vi "IR_OPO_Capture_V2.vi"(0 "Commands array":string[][](array[string])=[["Group20.825", "Group20.671", "Group20.814", "Group30.121"], ["Group2-0.528", "Group2-1.243", "Group2-0.539", "Group30.121"], ["Group20.374", "Group21.573", "Group20.363", "Group30.121"], ["Group2-0.242", "Group2-1.815", "Group2-0.253", "Group30.121"], ["Group20.165", "Group21.991", "Group20.154", "Group30.121"], ["Group2-0.077", "Group2-2.145", "Group2-0.088", "Group30.121"], ["Group20.044", "Group22.233", "Group20.033", "Group30.121"], ["Group2-2.310", "WT10", "WT10", "Group30.121"], ["Group22.310", "WT10", "WT10", "Group30.121"], ["Group2-2.310", "WT10", "WT10", "Group30.121"], ["Group22.310", "WT10", "WT10", "Group30.121"], ["Group2-2.310", "WT10", "WT10", "Group30.121"], ["Group22.310", "WT10", "WT10", "Group30.121"], ["Group2-0.011", "Group2-2.277", "Group2-0.022", "Group30.121"], ["Group20.066", "Group22.189", "Group20.055", "Group30.121"], ["Group2-0.121", "Group2-2.057", "Group2-0.132", "Group30.121"], ["Group20.209", "Group21.903", "Group20.198", "Group30.121"], ["Group2-0.297", "Group2-1.705", "Group2-0.308", "Group30.121"], ["Group20.451", "Group21.419", "Group20.440", "Group30.121"], ["Group2-0.660", "Group2-0.979", "Group2-0.671", "Group30.121"]], 1 "Laser on/off array":bool[][](array[boolean])=[[FALSE, TRUE, FALSE, FALSE], [FALSE, TRUE, FALSE, FALSE], [FALSE, TRUE, FALSE, FALSE], [FALSE, TRUE, FALSE, FALSE], [FALSE, TRUE, FALSE, FALSE], [FALSE, TRUE, FALSE, FALSE], [FALSE, TRUE, FALSE, FALSE], [TRUE, FALSE, FALSE, FALSE], [TRUE, FALSE, FALSE, FALSE], [TRUE, FALSE, FALSE, FALSE], [TRUE, FALSE, FALSE, FALSE], [TRUE, FALSE, FALSE, FALSE], [TRUE, FALSE, FALSE, FALSE], [FALSE, TRUE, FALSE, FALSE], [FALSE, TRUE, FALSE, FALSE], [FALSE, TRUE, FALSE, FALSE], [FALSE, TRUE, FALSE, FALSE], [FALSE, TRUE, FALSE, FALSE], [FALSE, TRUE, FALSE, FALSE], [FALSE, TRUE, FALSE, FALSE]], 3 "AD status":bool, 4 "Axis 2":string="Group3", 5 "XPS_Address":string="192.168.254.254", 6 "Axis 1":string="Group2", 7 "laser array index":i32, 8 "OPO on?":bool, 9 "Process time":dbl format="%#_13g", 11 "Axis Speed":dbl=1.0 format="%#_13g", 12 "stop":bool, 13 "Axis Initial Parameters":T1={"Velocity (units/seconds)"=1.0, "Acceleration (units/seconds²)"=20.0, "Minimum Jerk Time (seconds)"=0.005, "Maximum Jerk Time (seconds)"=0.009} {"Maximum Jerk Time (seconds)" format="%.6e"; "Minimum Jerk Time (seconds)" format="%.6e"; "Acceleration (units/seconds²)" format="%.6e"; "Velocity (units/seconds)" format="%.6e"}, 14 "ROI Area \n(mm2)":dbl=4.035870075999999, 15 "Acceleration (units/seconds²)":dbl=20.0) -> (2 "Elapsed time":dbl)   [LabVIEW 2016]
uses:
  case selector.ctl
panel:
  out "Capture Log":string
  out "Axis 1 position":dbl format="%.10f"
  out "Axis 2 position":dbl format="%.10f"
  out "Initial time":timestamp
  in  "Active Positioner":string
  out "Current Line":i32
  out "1D Laser Array":bool[](array[boolean])=[FALSE, TRUE, FALSE, FALSE, FALSE, TRUE, FALSE, FALSE, FALSE, TRUE, FALSE, FALSE, FALSE, TRUE, FALSE, FALSE, FALSE, TRUE, FALSE, FALSE, FALSE, TRUE, FALSE, FALSE, FALSE, TRUE, FALSE, FALSE, TRUE, FALSE, FALSE, FALSE, TRUE, FALSE, FALSE, FALSE, TRUE, FALSE, FALSE, FALSE, TRUE, FALSE, FALSE, FALSE, TRUE, FALSE, FALSE, FALSE, TRUE, FALSE, FALSE, FALSE, FALSE, TRUE, FALSE, FALSE, FALSE, TRUE, FALSE, FALSE, FALSE, TRUE, FALSE, FALSE, FALSE, TRUE, FALSE, FALSE, FALSE, TRUE, FALSE, FALSE, FALSE, TRUE, FALSE, FALSE, FALSE, TRUE, FALSE, FALSE]
  out "1D command array":string[](array[string])=["Group20.825", "Group20.671", "Group20.814", "Group30.121", "Group2-0.528", "Group2-1.243", "Group2-0.539", "Group30.121", "Group20.374", "Group21.573", "Group20.363", "Group30.121", "Group2-0.242", "Group2-1.815", "Group2-0.253", "Group30.121", "Group20.165", "Group21.991", "Group20.154", "Group30.121", "Group2-0.077", "Group2-2.145", "Group2-0.088", "Group30.121", "Group20.044", "Group22.233", "Group20.033", "Group30.121", "Group2-2.310", "WT10", "WT10", "Group30.121", "Group22.310", "WT10", "WT10", "Group30.121", "Group2-2.310", "WT10", "WT10", "Group30.121", "Group22.310", "WT10", "WT10", "Group30.121", "Group2-2.310", "WT10", "WT10", "Group30.121", "Group22.310", "WT10", "WT10", "Group30.121", "Group2-0.011", "Group2-2.277", "Group2-0.022", "Group30.121", "Group20.066", "Group22.189", "Group20.055", "Group30.121", "Group2-0.121", "Group2-2.057", "Group2-0.132", "Group30.121", "Group20.209", "Group21.903", "Group20.198", "Group30.121", "Group2-0.297", "Group2-1.705", "Group2-0.308", "Group30.121", "Group20.451", "Group21.419", "Group20.440", "Group30.121", "Group2-0.660", "Group2-0.979", "Group2-0.671", "Group30.121"]
  out "Current Command":string
  out "Current laser element":bool
  out "Total lines":i32=80
  in  "Active Axis":string
  out "Laser on/off":bool
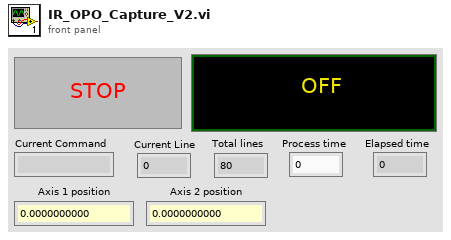
[diagram p1: front panel]
types:
  T1 = cluster{"Velocity (units/seconds)":dbl, "Acceleration (units/seconds²)":dbl, "Minimum Jerk Time (seconds)":dbl, "Maximum Jerk Time (seconds)":dbl}
  T2 = typedef "case selector.ctl" = enum16{"Initialize", "Element selection", "Laser", "Velocities", "Command", "Wait", "Exit"}
  T3 = enum16{"Initialize", "Lamp ON", "Lamp OFF", "Q-switch ON", "Q-switch OFF", "Adjust Energy", "Change Rep. Rate", "Send String"}
  T4 = enum16{"open", "replace", "create", "open or create", "replace or create", "replace or create with confirmation"}
  T5 = cluster{"connection TCP":refnum<k5>, "LogTo File":bool, "Log File refnum":refnum<file>, "no error if error log":bool}
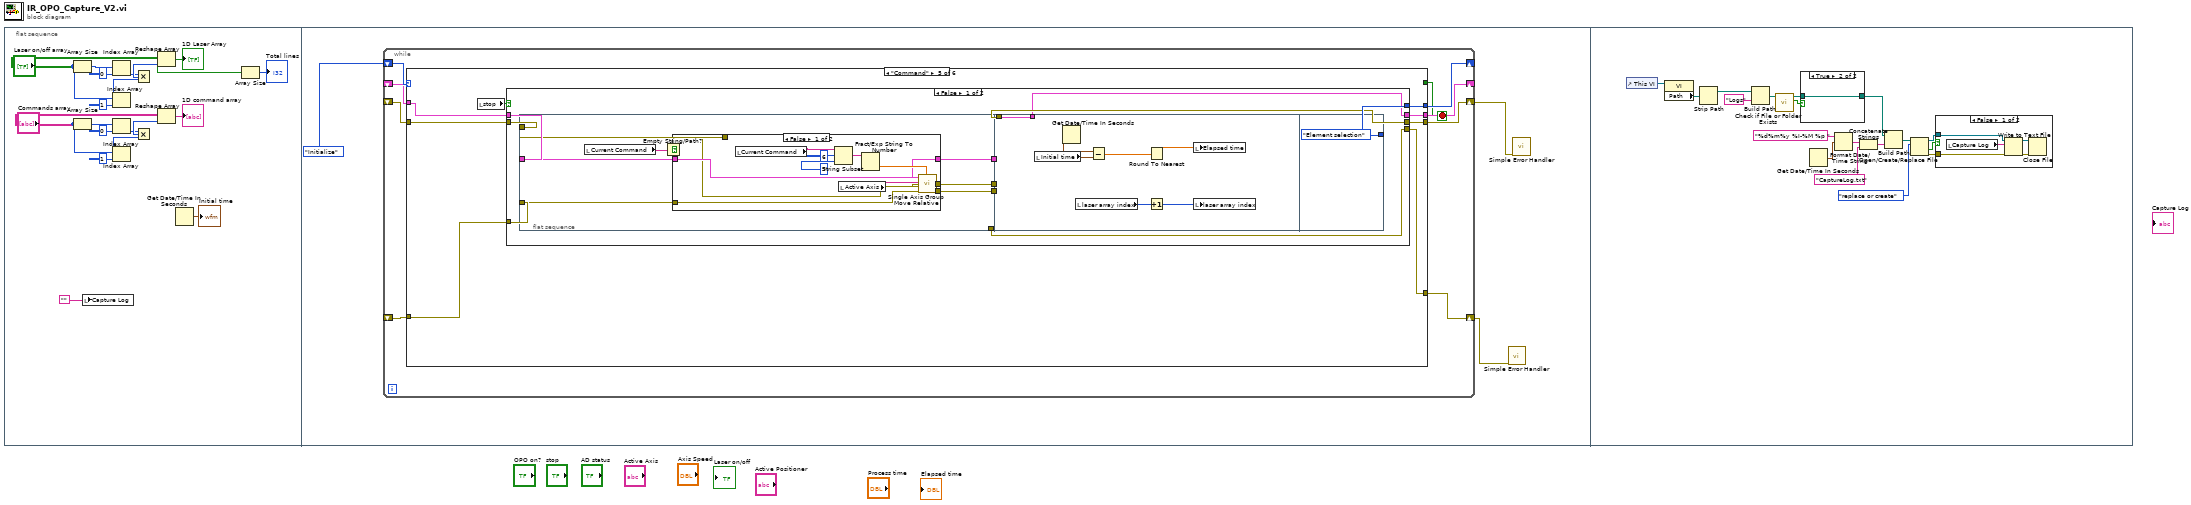
[diagram p0: block diagram]
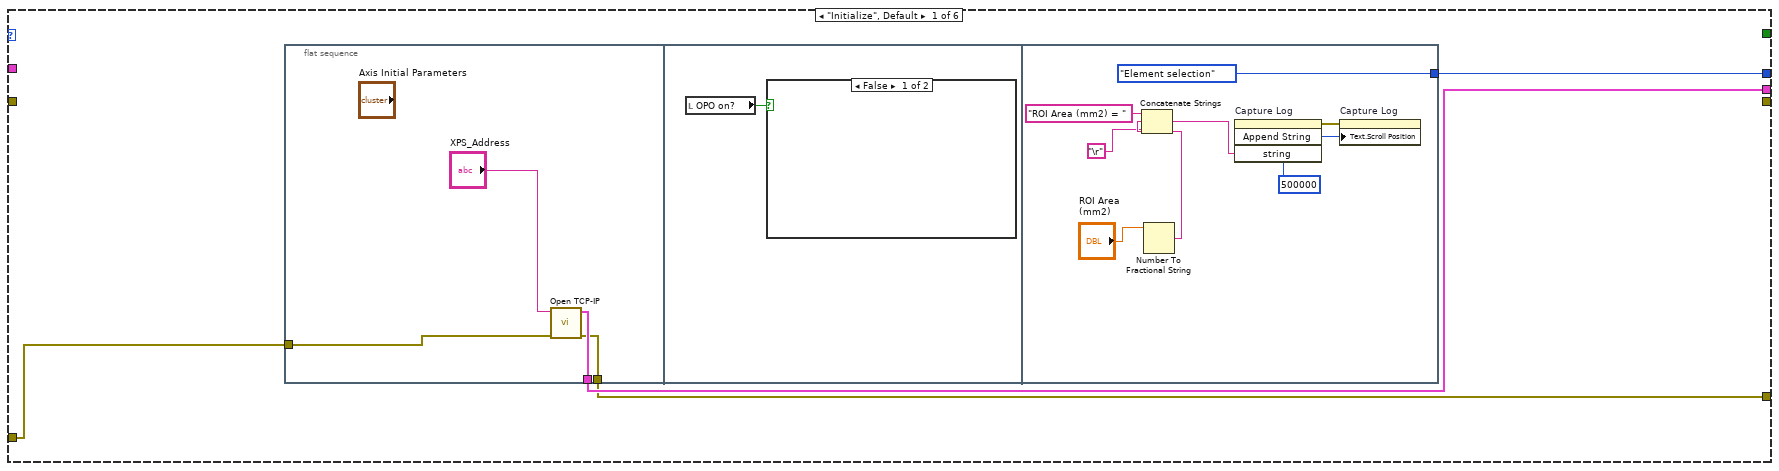
[diagram p2: hidden frame]
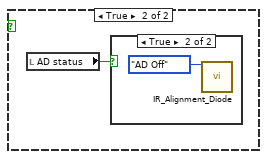
[diagram p3: hidden frame]
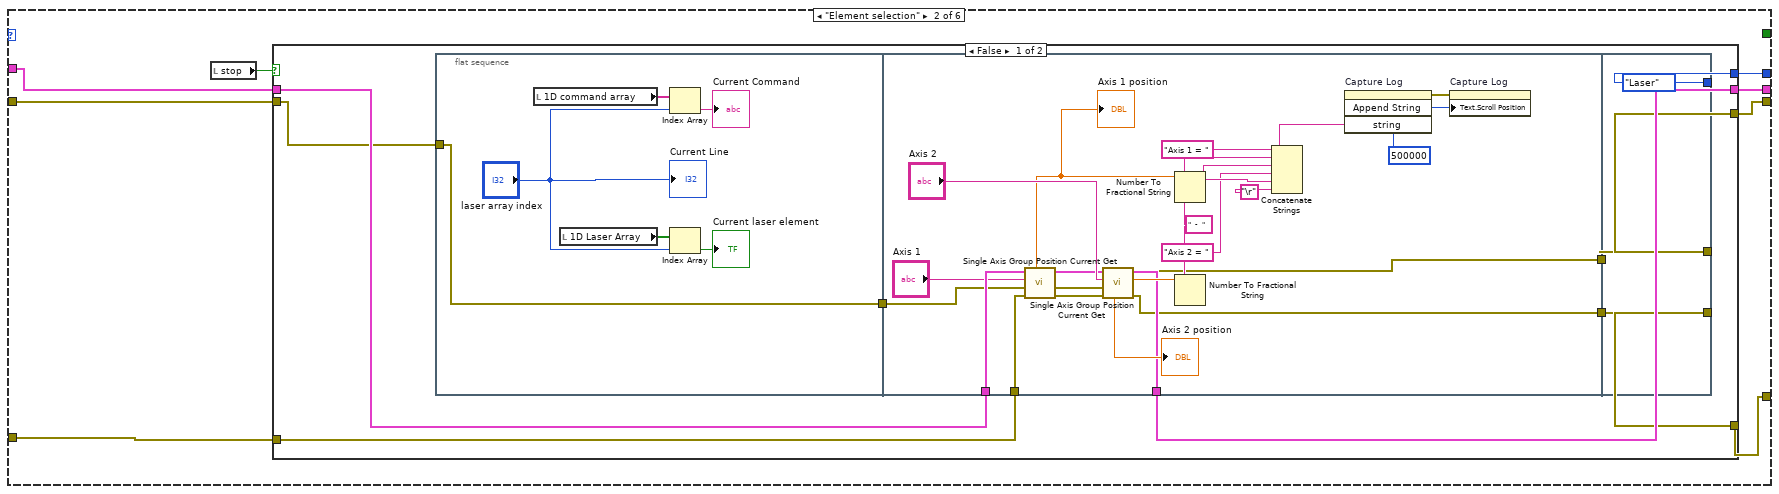
[diagram p5: hidden frame]
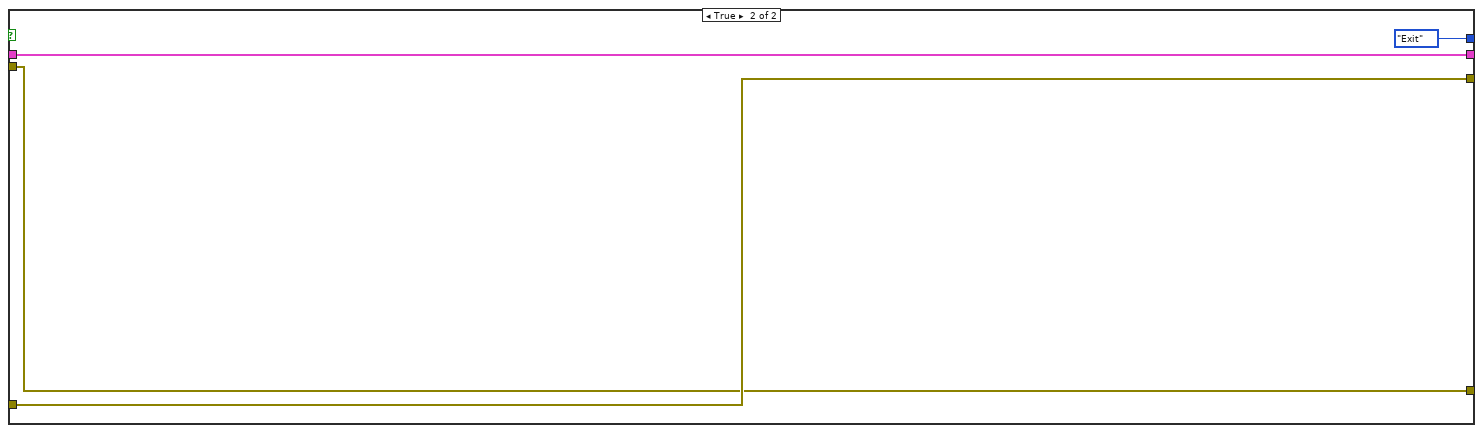
[diagram p6: hidden frame]
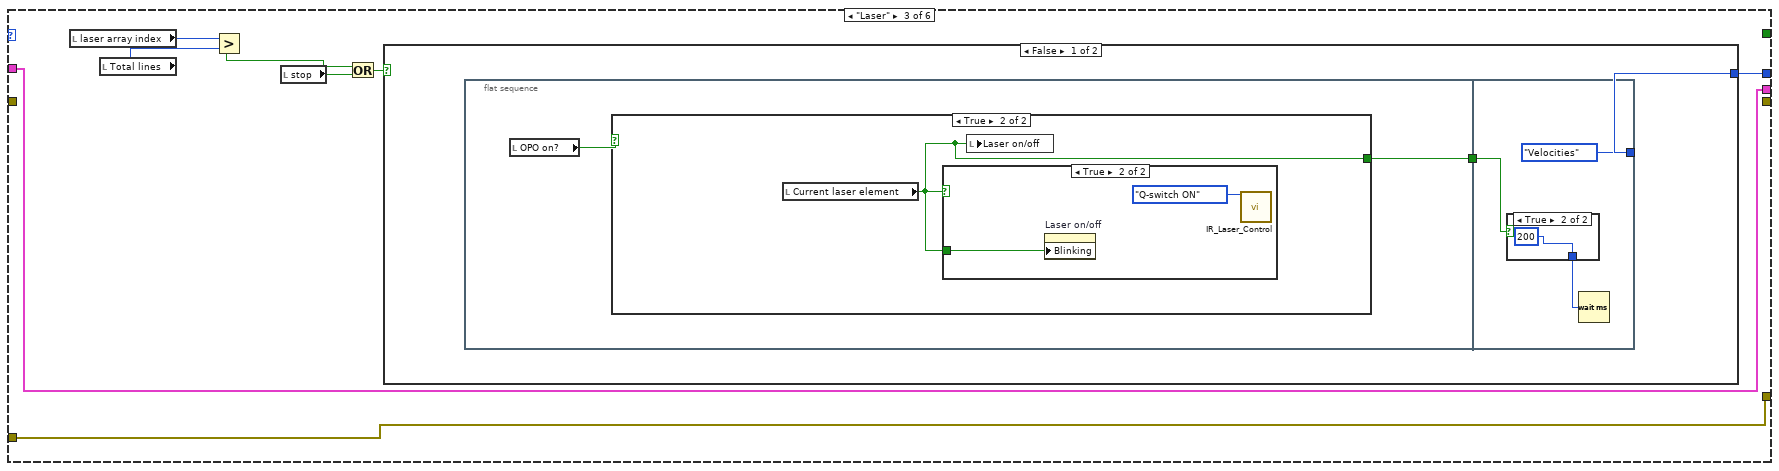
[diagram p7: hidden frame]
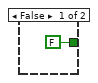
[diagram p8: hidden frame]
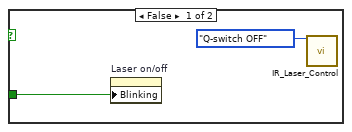
[diagram p9: hidden frame]
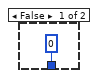
[diagram p10: hidden frame]
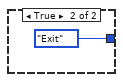
[diagram p11: hidden frame]
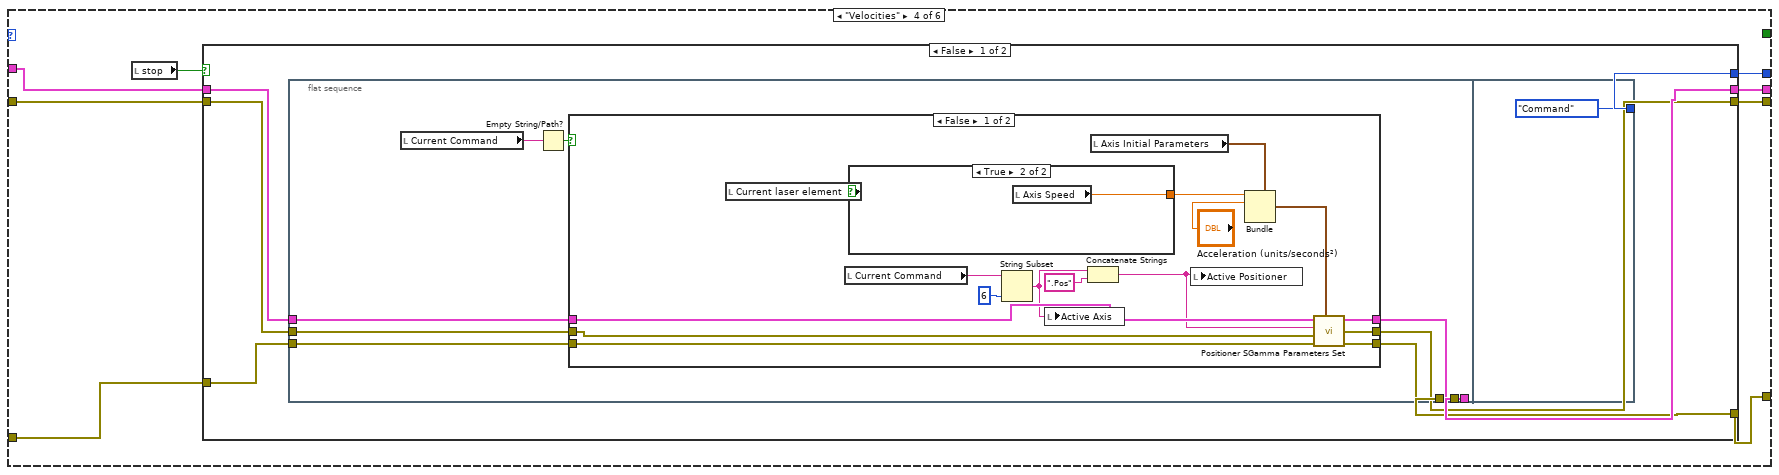
[diagram p12: hidden frame]
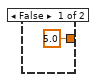
[diagram p13: hidden frame]
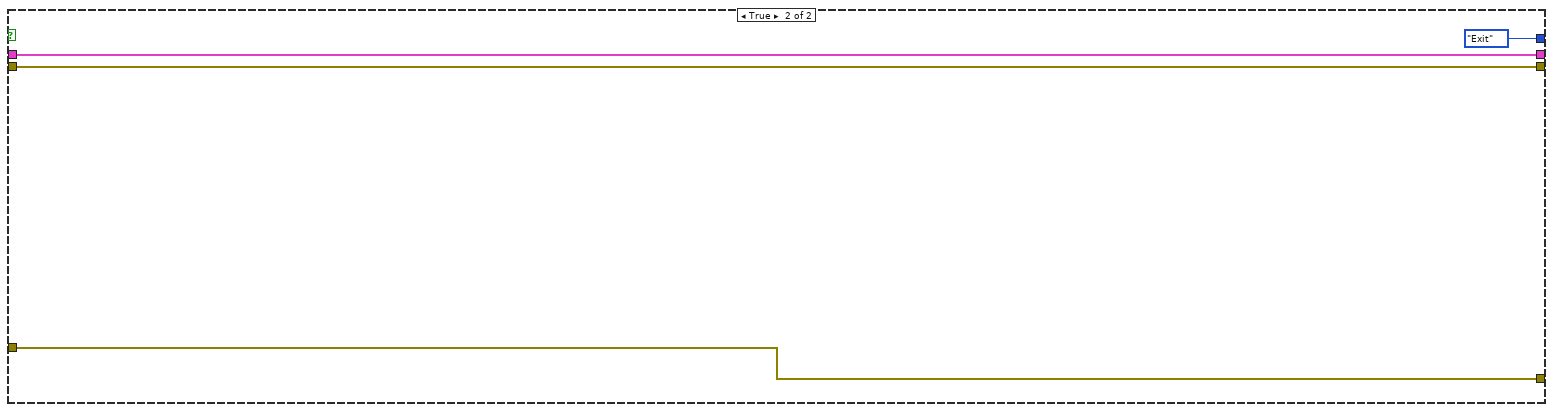
[diagram p15: hidden frame]
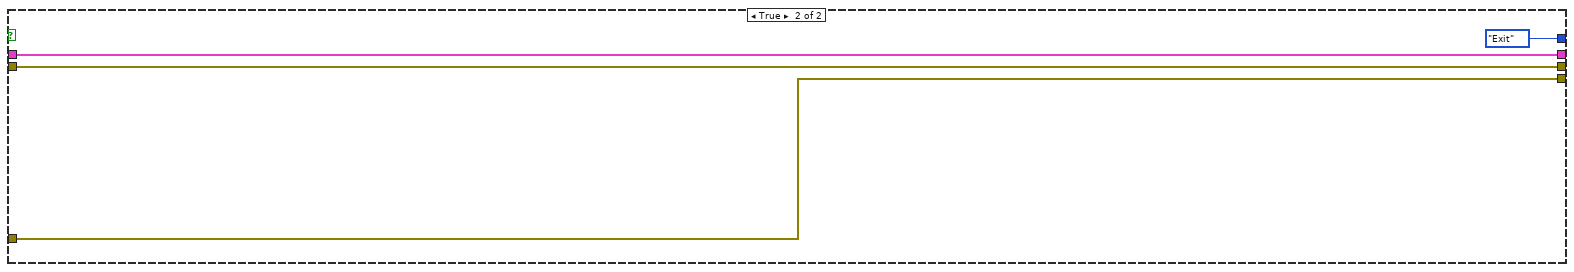
[diagram p17: hidden frame]
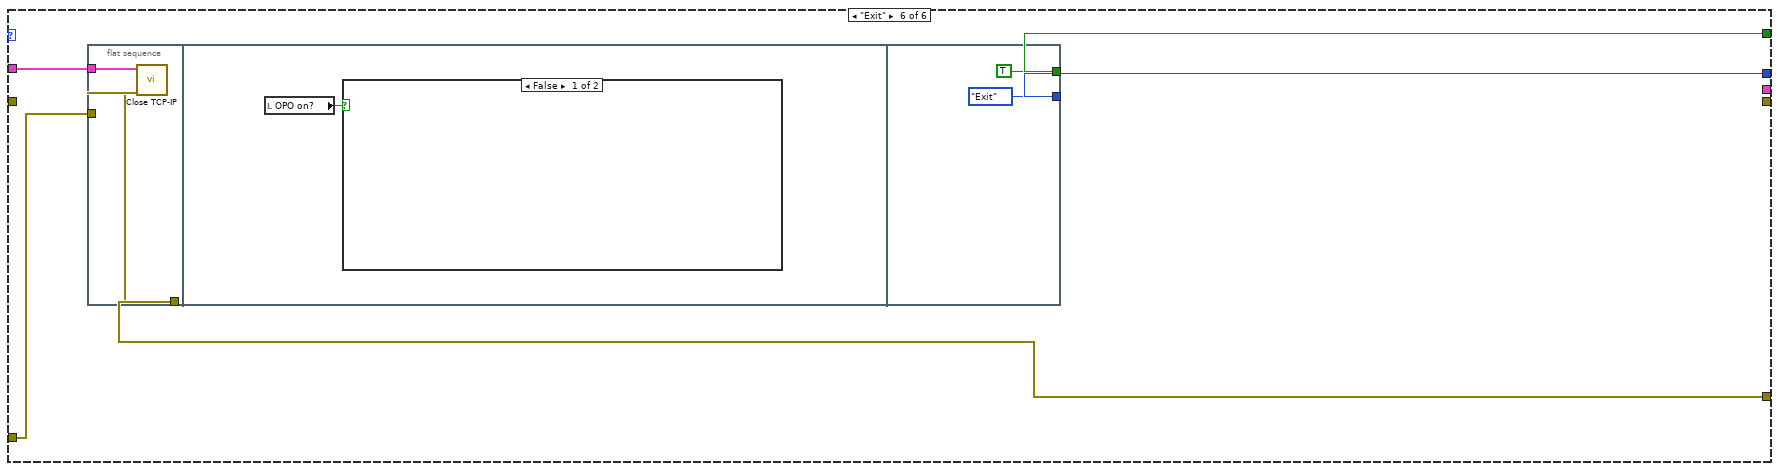
[diagram p18: hidden frame]
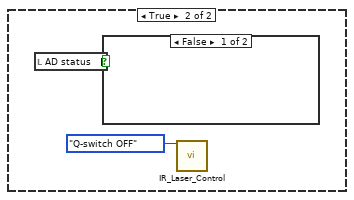
[diagram p19: hidden frame]
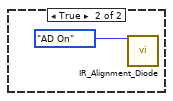
[diagram p20: hidden frame]
diagram:
  n1 = flat-sequence {
    frame #0 {
      n2 = Array Size(array="Laser on/off array") -> (size(s)=w11:i32[])
      n3 = Array Size(array="Commands array") -> (size(s)=w3:i32[])
      n4 = local write "Capture Log"("") -> ()
      n5 = Index Array(array=w11, index=0) -> (element=w14:i32)
      n6 = Index Array(array=w11, index=1) -> (element=w15:i32)
      n7 = Index Array(array=w3, index=0) -> (element=w6:i32)
      n8 = Index Array(array=w3, index=1) -> (element=w7:i32)
      n9 = Multiply(x=w14, y=w15) -> (x*y=w16:i32)
      n10 = Multiply(x=w6, y=w7) -> (x*y=w8:i32)
      n11 = Reshape Array("Laser on/off array", w16) -> (w19:bool[])
      "1D Laser Array" <- w19
      n12 = Reshape Array("Commands array", w8) -> (→"1D command array":string[])
      n13 = Get Date/Time In Seconds() -> (seconds since 1Jan1904=→"Initial time":timestamp)
      n14 = Array Size(array=w19) -> (size(s)=→"Total lines":i32)
    }
    frame #1 {
      n15 = while {
        shift-right: [w30] -> _
        shift-left: case_selector."Initialize" -> [w31]
        shift-right: [w28] -> w20
        shift-left: _ -> [w29]
        shift-right: [w27] -> _
        shift-left: _ -> [w26]
        shift-right: [w25] -> w21
        shift-left: _ -> [w24]
        stop <- w23 stop-if-true
        n16 = case shown="\"Command\"" w31 {
          tunnel: [w35 w58 w111 w135 w184 w233] -> w30
          tunnel: w29 -> [w34 w55 w110 w133 w182 w234]
          tunnel: [w32 w52 w110 w132 w181 w232] -> w28
          tunnel: [w33 w51 w104 w130 w179 _] -> w27
          tunnel: w26 -> [_ w56 w104 w131 w180 w231]
          tunnel: [_ w53 _ w129 w177 _] -> w25
          tunnel: w24 -> [_ w54 _ w128 w178 _]
          tunnel: [_ _ _ _ _ w230] -> w23
          frame "Initialize", Default {
            n17 = flat-sequence {
              tunnel: w34 -> [w38]
              tunnel: [w37] -> w33
              tunnel: [w36] -> w32
              tunnel: [case_selector."Element selection"] -> w35
              frame #0 {
                n18 = call <userlib>:"Open TCP-IP.vi"("error in (no error)"=w38, "IP address"="XPS_Address") -> ("error out"=w36:errorcluster, "Connection ID"=w37:T5)  [unwired: 7 in, 1 out]
              }
              frame #1 {
                n19 = local read "OPO on?"() -> (w40:bool)
                n20 = case shown="False" w40 {
                  frame False {
                  }
                  frame True {
                    n21 = local read "AD status"() -> (w41:bool)
                    n22 = case shown="True" w41 {
                      frame False {
                      }
                      frame True {
                        n23 = call "IR_Alignment_Diode.vi"("AD Action"=enum16{"AD Off", "AD On"}."AD Off") -> ()  [unwired: 14 in, 1 out]
                      }
                    }
                  }
                }
              }
              frame #2 {
                n24 = Number To Fractional String(number="ROI Area \n(mm2)") -> (F-format string=w46:string)  [unwired: 3 in]
                n25 = Concatenate Strings("ROI Area (mm2) = " ("string"), w46, "\r") -> (w44:string)
                n26 = invoke on="Capture Log" class="Str" method="Append String"("string"=w44) -> (error out=w48:errorcluster)  [unwired: 3 in, 3 out]
                n27 = property on="Capture Log" class="Str"(error in=w48, "Text.Scroll Position"=u32 500000) -> ()  [unwired: 1 in, 2 out]
              }
            }
          }
          frame "Element selection" {
            n28 = local read "stop"() -> (w57:bool)
            n29 = case shown="False" w57 {
              tunnel: [w67 case_selector."Exit"] -> w58
              tunnel: w56 -> [w68 w102]
              tunnel: w55 -> [w61 w101]
              tunnel: w54 -> [w60 w100]
              tunnel: [w62 w101] -> w53
              tunnel: [w64 w100] -> w52
              tunnel: [w66 w102] -> w51
              frame False {
                n30 = flat-sequence {
                  tunnel: w60 -> [w69]
                  tunnel: [w69] -> w59
                  tunnel: w68 -> [w87]
                  tunnel: w61 -> [w85]
                  tunnel: [w78] -> w66
                  tunnel: [w77] -> w65
                  tunnel: [w76] -> w63
                  tunnel: w59 -> [w75]
                  tunnel: [case_selector."Laser"] -> w67
                  tunnel: w65 -> [w98]
                  tunnel: [w98] -> w64
                  tunnel: w63 -> [w97]
                  tunnel: [w97] -> w62
                  frame #0 {
                    n31 = local read "1D command array"() -> (w72:string[])
                    n32 = local read "1D Laser Array"() -> (w71:bool[])
                    n33 = Index Array(array=w72, index="laser array index") -> (element=→"Current Command":string)
                    n34 = Index Array(array=w71, index="laser array index") -> (element=→"Current laser element":bool)
                    "Current Line" <- "laser array index"
                  }
                  frame #1 {
                    n35 = call <userlib>:"Single Axis Group Position Current Get.vi"("error in (no error)"=w85, "XPS error in (no error)"=w75, "SingleAxis Group  Name (250 c max)"="Axis 1", "connection ID in"=w87) -> ("error out"=w79:errorcluster, "XPS error out"=w80:errorcluster, "Current Position (units)"=w84:dbl, "connection ID out"=w81:T5)  [unwired: 4 in]
                    "Axis 1 position" <- w84
                    n36 = call <userlib>:"Single Axis Group Position Current Get.vi"("error in (no error)"=w79, "XPS error in (no error)"=w80, "SingleAxis Group  Name (250 c max)"="Axis 2", "connection ID in"=w81) -> ("error out"=w77:errorcluster, "XPS error out"=w76:errorcluster, "Current Position (units)"=w83:dbl, "connection ID out"=w78:T5)  [unwired: 4 in]
                    "Axis 2 position" <- w83
                    n37 = Number To Fractional String(number=w84) -> (F-format string=w95:string)  [unwired: 3 in]
                    n38 = Number To Fractional String(number=w83) -> (F-format string=w93:string)  [unwired: 3 in]
                    n39 = Concatenate Strings("Axis 1 = " ("string"), w95, "  -  " ("string"), "Axis 2 = " ("string"), w93, "\r") -> (w90:string)
                    n40 = invoke on="Capture Log" class="Str" method="Append String"("string"=w90) -> (error out=w89:errorcluster)  [unwired: 3 in, 3 out]
                    n41 = property on="Capture Log" class="Str"(error in=w89, "Text.Scroll Position"=u32 500000) -> ()  [unwired: 1 in, 2 out]
                  }
                  frame #2 {
                  }
                }
              }
              frame True {
              }
            }
          }
          frame "Laser" {
            n42 = local read "laser array index"() -> (w108:i32)
            n43 = local read "Total lines"() -> (w109:i32)
            n44 = Greater?(x=w108, y=w109) -> (0:w106:bool)
            n45 = local read "stop"() -> (w107:bool)
            n46 = Or(x=w106, y=w107) -> (x .or. y?=w105:bool)
            n47 = case shown="False" w105 {
              tunnel: [w113 case_selector."Exit"] -> w111
              frame False {
                n48 = flat-sequence {
                  tunnel: [w114] -> w112
                  tunnel: [case_selector."Velocities"] -> w113
                  tunnel: w112 -> [w123]
                  frame #0 {
                    n49 = local read "OPO on?"() -> (w115:bool)
                    n50 = case shown="True" w115 {
                      tunnel: [FALSE ("Current laser element") w117] -> w114
                      frame False {
                      }
                      frame True {
                        n51 = local read "Current laser element"() -> (w117:bool)
                        n52 = case shown="True" w117 {
                          tunnel: w117 -> [w118 w120]
                          frame False {
                            n53 = property on="Laser on/off" class="Bool (strict)"("Blinking"=w118) -> ()  [unwired: 2 in, 2 out]
                            n54 = call "IR_Laser_Control.vi"("Action"=T3."Q-switch OFF") -> ()  [unwired: 14 in, 1 out]
                          }
                          frame True {
                            n55 = property on="Laser on/off" class="Bool (strict)"("Blinking"=w120) -> ()  [unwired: 2 in, 2 out]
                            n56 = call "IR_Laser_Control.vi"("Action"=T3."Q-switch ON") -> ()  [unwired: 14 in, 1 out]
                          }
                        }
                        n57 = local write "Laser on/off"(w117) -> ()
                      }
                    }
                  }
                  frame #1 {
                    n58 = case shown="True" w123 {
                      tunnel: [u32 0 ("milliseconds to wait") u32 200 ("milliseconds to wait")] -> w122
                      frame False {
                      }
                      frame True {
                      }
                    }
                    n59 = Wait (ms)(milliseconds to wait=w122) -> ()  [unwired: 1 out]
                  }
                }
              }
              frame True {
              }
            }
          }
          frame "Velocities" {
            n60 = local read "stop"() -> (w134:bool)
            n61 = case shown="False" w134 {
              tunnel: [w142 case_selector."Exit"] -> w135
              tunnel: w133 -> [w141 w175]
              tunnel: [w138 w175] -> w132
              tunnel: w131 -> [w140 w174]
              tunnel: [w139 w174] -> w130
              tunnel: [w137 w173] -> w129
              tunnel: w128 -> [w136 w173]
              frame False {
                n62 = flat-sequence {
                  tunnel: w141 -> [w148]
                  tunnel: w140 -> [w150]
                  tunnel: [w149] -> w139
                  tunnel: [w147] -> w138
                  tunnel: [w146] -> w137
                  tunnel: w136 -> [w145]
                  tunnel: [case_selector."Command"] -> w142
                  frame #0 {
                    n63 = local read "Current Command"() -> (w144:string)
                    n64 = Empty String/Path?(string/path=w144) -> (empty?=w143:bool)
                    n65 = case shown="False" w143 {
                      tunnel: w150 -> [w163 w169]
                      tunnel: [w162 w169] -> w149
                      tunnel: w148 -> [w161 w170]
                      tunnel: [w160 w170] -> w147
                      tunnel: [w155 w171] -> w146
                      tunnel: w145 -> [w154 w171]
                      frame False {
                        n66 = local read "Current laser element"() -> (w166:bool)
                        n67 = local read "Current Command"() -> (w164:string)
                        n68 = case shown="True" w166 {
                          tunnel: [5.0 w168] -> w159
                          frame False {
                          }
                          frame True {
                            n69 = local read "Axis Speed"() -> (w168:dbl)
                          }
                        }
                        n70 = String Subset(string=w164, length (rest)=6 ("length (rest)")) -> (substring=w153:string)  [unwired: 1 in]
                        n71 = local write "Active Axis"(w153) -> ()
                        n72 = Concatenate Strings(w153, ".Pos" ("string")) -> (w152:string)
                        n73 = local read "Axis Initial Parameters"() -> (w157:T1)
                        n74 = local write "Active Positioner"(w152) -> ()
                        n75 = Bundle(cluster=w157, "Velocity (units/seconds)"=w159, "Acceleration (units/seconds²)"="Acceleration (units/seconds²)") -> (w158:T1)  [unwired: 2 in]
                        n76 = call <userlib>:"Positioner SGamma Parameters Set.vi"("SGamma Parameters"=w158, "error in (no error)"=w161, "XPS error in (no error)"=w154, "Positioner Name (250 c max)"=w152, "connection ID in"=w163) -> ("error out"=w160:errorcluster, "XPS error out"=w155:errorcluster, "connection ID out"=w162:T5)  [unwired: 4 in]
                      }
                      frame True {
                      }
                    }
                  }
                  frame #1 {
                  }
                }
              }
              frame True {
              }
            }
          }
          frame "Command" {
            n77 = local read "stop"() -> (w183:bool)
            n78 = case shown="False" w183 {
              tunnel: [w188 case_selector."Exit"] -> w184
              tunnel: w182 -> [w192 w228]
              tunnel: [w186 w228] -> w181
              tunnel: w180 -> [w194 w227]
              tunnel: [w185 w227] -> w179
              tunnel: w178 -> [w191 w226]
              tunnel: [w187 w226] -> w177
              frame False {
                n79 = flat-sequence {
                  tunnel: w194 -> [w202]
                  tunnel: [w201] -> w193
                  tunnel: w192 -> [w198]
                  tunnel: w191 -> [w197]
                  tunnel: [w196] -> w190
                  tunnel: [w195] -> w189
                  tunnel: w193 -> [w216]
                  tunnel: w190 -> [w218]
                  tunnel: w189 -> [w217]
                  tunnel: [w218] -> w187
                  tunnel: [w217] -> w186
                  tunnel: [w216] -> w185
                  tunnel: [case_selector."Element selection"] -> w188
                  frame #0 {
                    n80 = local read "Current Command"() -> (w199:string)
                    n81 = Empty String/Path?(string/path=w199) -> (empty?=w200:bool)
                    n82 = case shown="False" w200 {
                      tunnel: w202 -> [w214 w215]
                      tunnel: [w207 w215] -> w201
                      tunnel: w198 -> [w206 _]
                      tunnel: w197 -> [w205 _]
                      tunnel: [w204 _] -> w196
                      tunnel: [w203 _] -> w195
                      frame False {
                        n83 = local read "Current Command"() -> (w213:string)
                        n84 = String Subset(string=w213, offset (0)=6, length (rest)=9 ("length (rest)")) -> (substring=w210:string)
                        n85 = local read "Active Axis"() -> (w208:string)
                        n86 = Fract/Exp String To Number(string=w210) -> (number=w209:dbl)  [unwired: 3 in, 1 out]
                        n87 = call <userlib>:"Single Axis Group Move Relative.vi"("Target Displacement (units)"=w209, "error in (no error)"=w206, "XPS error in (no error)"=w205, "SingleAxis Group  Name (250 c max)"=w208, "connection ID in"=w214) -> ("error out"=w203:errorcluster, "XPS error out"=w204:errorcluster, "connection ID out"=w207:T5)  [unwired: 4 in]
                      }
                      frame True {
                      }
                    }
                  }
                  frame #1 {
                    n88 = local read "Initial time"() -> (w221:timestamp)
                    n89 = Get Date/Time In Seconds() -> (seconds since 1Jan1904=w222:timestamp)
                    n90 = local read "laser array index"() -> (w224:i32)
                    n91 = Subtract(x=w222, y=w221) -> (x-y=w220:dbl)
                    n92 = Round To Nearest(number=w220) -> (nearest integer value=w219:dbl)
                    n93 = Increment(x=w224) -> (x+1=w223:i32)
                    n94 = local write "Elapsed time"(w219) -> ()
                    n95 = local write "laser array index"(w223) -> ()
                  }
                  frame #2 {
                  }
                }
              }
              frame True {
              }
            }
          }
          frame "Exit" {
            n96 = flat-sequence {
              tunnel: w234 -> [w236]
              tunnel: [w235] -> w232
              tunnel: w231 -> [w237]
              tunnel: [case_selector."Exit"] -> w233
              tunnel: [TRUE] -> w230
              frame #0 {
                n97 = call <userlib>:"Close TCP-IP.vi"("error in (no error)"=w236, "connection ID in"=w237) -> ("Error out"=w235:errorcluster)  [unwired: 9 in]
              }
              frame #1 {
                n98 = local read "OPO on?"() -> (w238:bool)
                n99 = case shown="False" w238 {
                  frame False {
                  }
                  frame True {
                    n100 = local read "AD status"() -> (w239:bool)
                    n101 = case shown="False" w239 {
                      frame False {
                      }
                      frame True {
                        n102 = call "IR_Alignment_Diode.vi"("AD Action"=enum16{"AD Off", "AD On"}."AD On") -> ()  [unwired: 14 in, 1 out]
                      }
                    }
                    n103 = call "IR_Laser_Control.vi"("Action"=T3."Q-switch OFF") -> ()  [unwired: 14 in, 1 out]
                  }
                }
              }
              frame #2 {
              }
            }
          }
        }
      }
      n104 = call <vilib>:"Simple Error Handler.vi"("error in (no error)"=w20) -> ()  [unwired: 4 in, 5 out]
      n105 = call <vilib>:"Simple Error Handler.vi"("error in (no error)"=w21) -> ()  [unwired: 4 in, 5 out]
    }
    frame #2 {
      n106 = control-ref of="This VI"() -> (w261:refnum<vi>)
      n107 = property class="VI"(reference=w261) -> ("Path"=w260:path)  [unwired: 1 in, 2 out]
      n108 = Strip Path(path=w260) -> (stripped path=w251:path)  [unwired: 1 out]
      n109 = Build Path(base path=w251, name or relative path="Logs") -> (appended path=w253:path)
      n110 = call <vilib>:"Check if File or Folder Exists.vi"("path"=w253) -> ("file or folder exists?"=w252:bool, "dup path"=w250:path)  [unwired: 8 in, 1 out]
      n111 = case shown="True" w252 {
        tunnel: w250 -> [w263 w264]
        tunnel: [w262 w264] -> w247
        frame False {
          n112 = Create Folder(path (use dialog)=w263) -> (created path=w262:path)  [unwired: 2 in, 2 out]
        }
        frame True {
        }
      }
      n113 = Get Date/Time In Seconds() -> (seconds since 1Jan1904=w256:timestamp)
      n114 = Format Date/Time String(time format string (%c)="%d%m%y %I-%M %p ", seconds (now)=w256) -> (date/time string=w258:string)  [unwired: 1 in]
      n115 = Concatenate Strings(w258, "CaptureLog.txt") -> (w248:string)
      n116 = Build Path(base path=w247, name or relative path=w248) -> (appended path=w249:path)
      n117 = Open/Create/Replace File(file path (use dialog)=w249, operation (0:open)=T4."replace or create") -> (refnum out=w246:refnum<file>, cancelled=w244:bool, error out=w245:errorcluster)  [unwired: 4 in]
      n118 = case shown="False" w244 {
        tunnel: w246 -> [w269 _]
        tunnel: w245 -> [w267 _]
        frame False {
          n119 = local read "Capture Log"() -> (w268:string)
          n120 = Write to Text File(file (use dialog)=w269, text=w268, error in=w267) -> (refnum out=w266:refnum<file>, error out=w265:errorcluster)  [unwired: 2 out]
          n121 = Close File(refnum=w266, error in=w265) -> ()  [unwired: 2 out]
        }
        frame True {
        }
      }
    }
  }
